vi "Zoe z function.vi"() -> ()   [LabVIEW 2014]
uses:
  <vilib>/vision/NI_Vision_Development_Module.lvlib
panel:
  out "Z Estimation":sgl(graph)
  out "Stage Position":dbl(graph)
  out "Segmented Particle":T1(plugin-control)
  out "COM Y":dbl(graph)
  out "COM X":dbl(graph)
  in  "Stage Position":dbl
  out "Cropped ROI":T1(plugin-control)
  in  "CrossCorrelation RADIUS":dbl
  in  "Template Path":path
  in  "Template Path  2":path
  out "Computational time (s)":dbl
  out "THIS ROI":T1(plugin-control)
  out "Original Image":T1(plugin-control)
  out "Y Centroid":sgl
  out "X Centroid":sgl
  in  "Reset Crop":bool
  in  "Crop":bool
  in  "ROI RADIUS":dbl
  in  "File Path":path
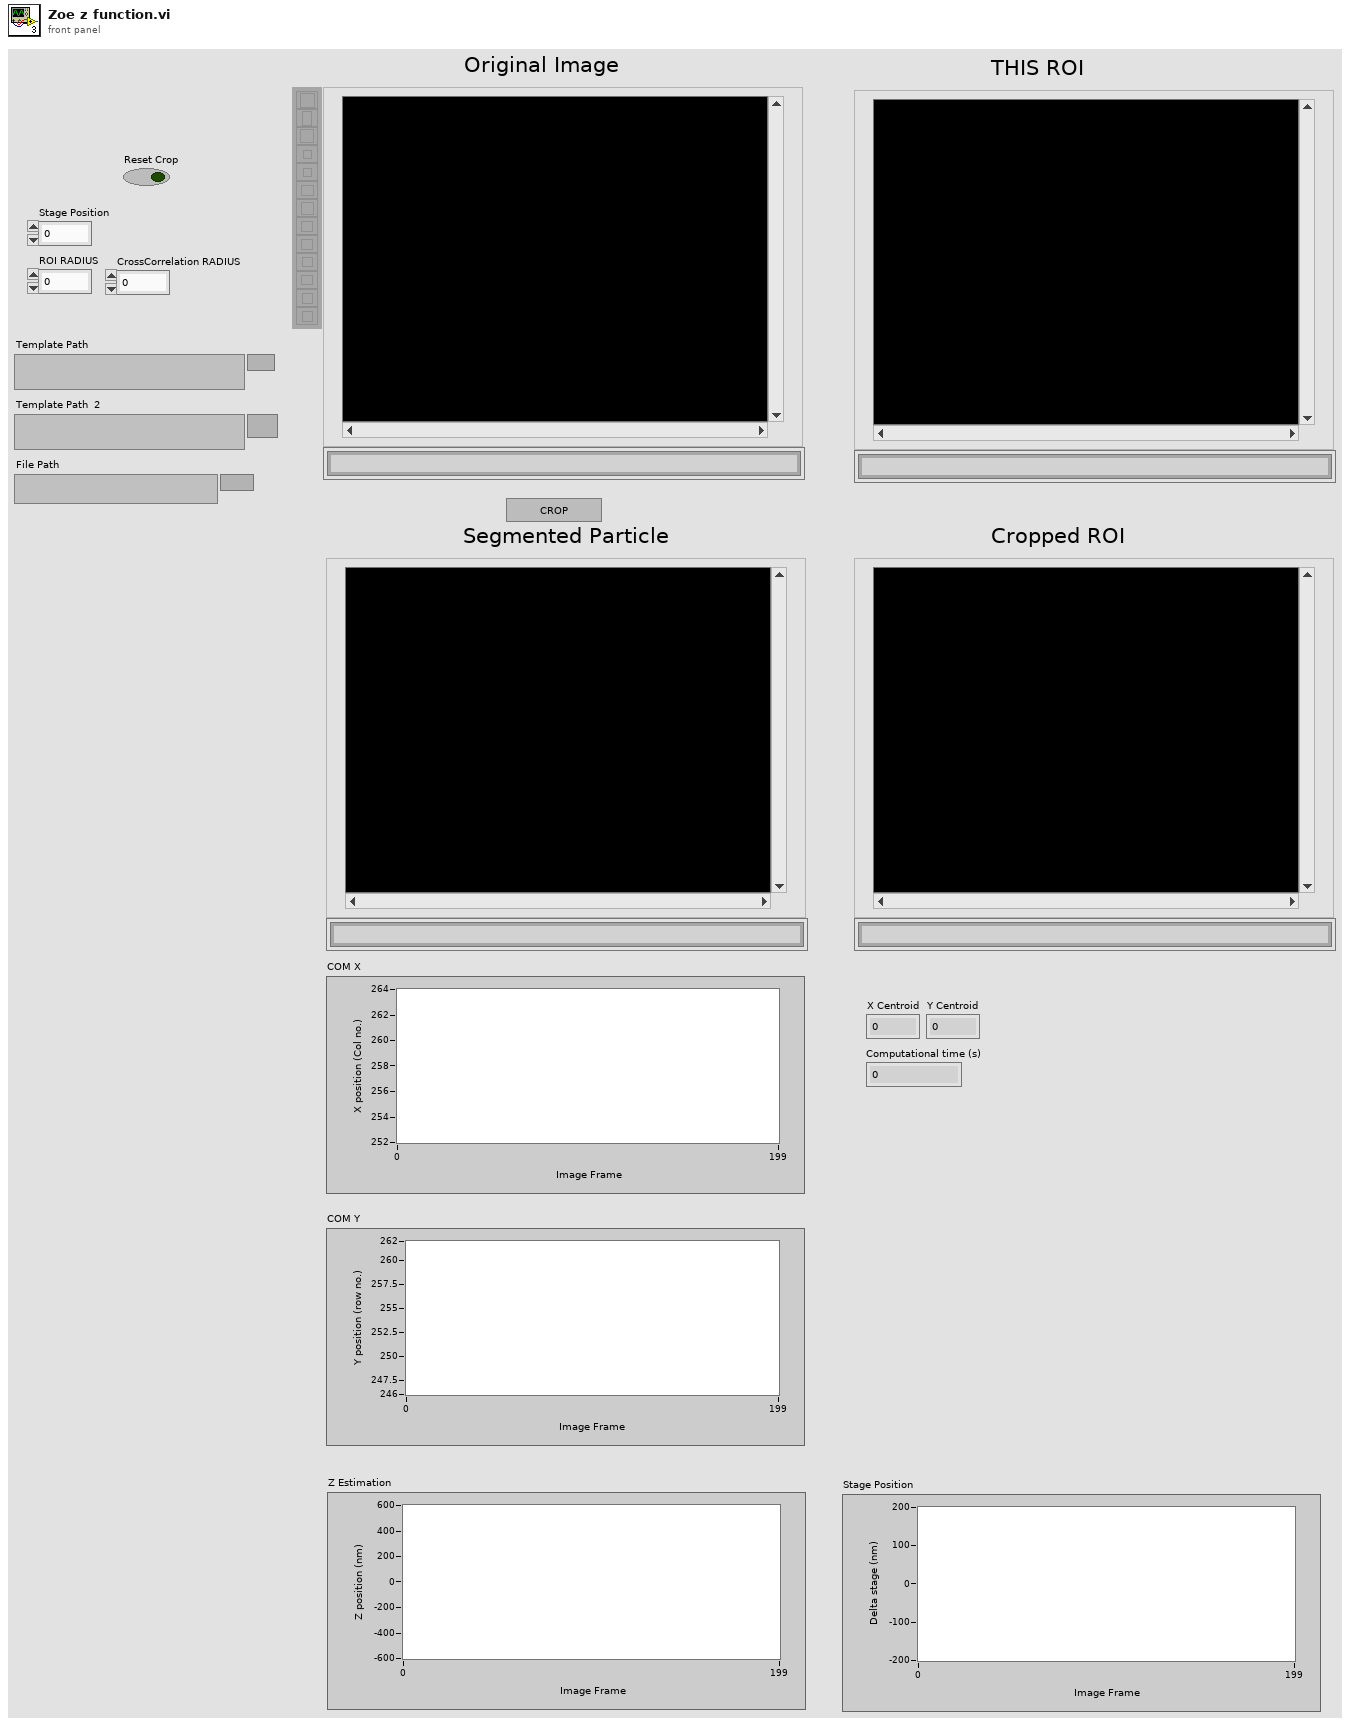
[diagram p1: front panel]
types:
  T1 = typedef "IMAQ Image.ctl" = refnum<image>
  T2 = typedef "Image Type" = u32
  T3 = cluster{"Global Rectangle":i32[], "Contours":cluster{"Contour Type":u32, "ROI Type":u32, "Points":i32[]}[]}
  T4 = typedef "IMAQ Rectangle" = cluster{"Left":i32, "Top":i32, "Right":i32, "Bottom":i32, "Rotation":dbl}
  T5 = cluster{"Mean Value":sgl, "Standard Variation":sgl, "Minimal Value":sgl, "Maximal Value":sgl, "Area (calibrated)":sgl, "Area (pixels)":u32, "%":sgl, "Calibration Valid":bool}
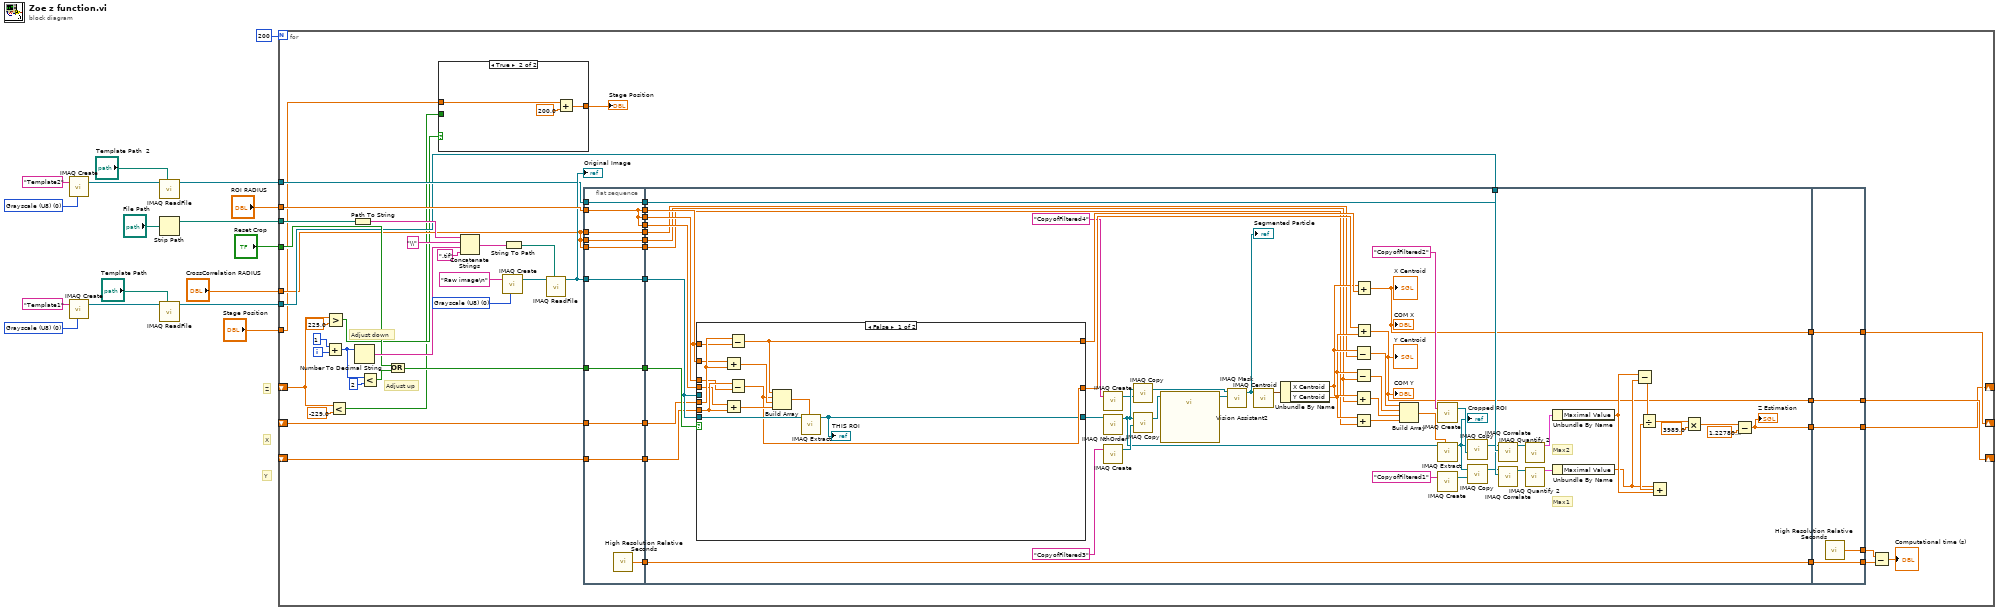
[diagram p0: block diagram]
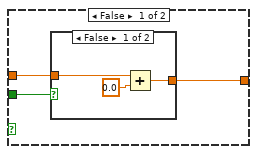
[diagram p2: hidden frame]
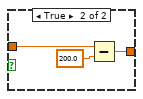
[diagram p3: hidden frame]
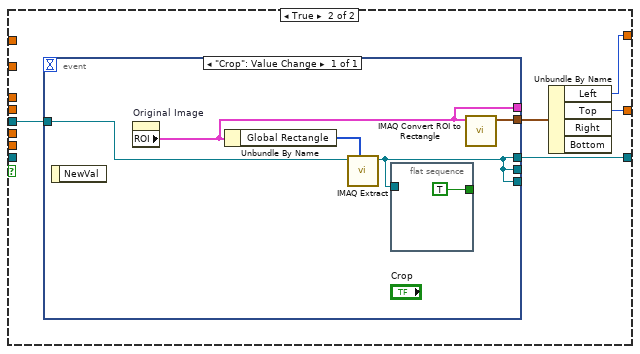
[diagram p4: hidden frame]
diagram:
  w4 = T2 0 items=["Grayscale (U8)", "Grayscale (I16)", "Grayscale (SGL)", "Complex (CSG)", "RGB (U32)", "HSL (U32)", "RGB (U64)", "Grayscale (U16)"] ("Image Type")
  w9 = T2 0 items=["Grayscale (U8)", "Grayscale (I16)", "Grayscale (SGL)", "Complex (CSG)", "RGB (U32)", "HSL (U32)", "RGB (U64)", "Grayscale (U16)"] ("Image Type")
  # "Z"
  # "X"
  # "Y"
  n1 = call "IMAQ Create"("Image Name"="Template2", "Image Type"=w9) -> ("New Image"=w11:T1)  [unwired: 3 in, 1 out]
  n2 = call "IMAQ Create"("Image Name"="Template1", "Image Type"=w4) -> ("New Image"=w6:T1)  [unwired: 3 in, 1 out]
  n3 = call "IMAQ ReadFile"("File Path"="Template Path  2", "Image"=w11) -> ("Image Out"=w8:T1)  [unwired: 5 in, 4 out]
  n4 = Strip Path(path="File Path") -> (stripped path=w14:path)  [unwired: 1 out]
  n5 = call "IMAQ ReadFile"("File Path"="Template Path", "Image"=w6) -> ("Image Out"=w3:T1)  [unwired: 5 in, 4 out]
  n6 = for {
    N: 200 -> [_]
    tunnel: "Reset Crop" -> [w41]
    shift-right: [w64] -> _
    shift-left: _ -> [w61]
    shift-right: [w66] -> _
    shift-left: _ -> [w59]
    tunnel: "ROI RADIUS" -> [w55]
    tunnel: w14 -> [w54]
    tunnel: w8 -> [w35]
    tunnel: w3 -> [w34]
    tunnel: "CrossCorrelation RADIUS" -> [w29]
    shift-right: [w20] -> _
    shift-left: _ -> [w24]
    tunnel: "Stage Position" -> [w21]
    i -> [w46]
    w48 = T2 0 items=["Grayscale (U8)", "Grayscale (I16)", "Grayscale (SGL)", "Complex (CSG)", "RGB (U32)", "HSL (U32)", "RGB (U64)", "Grayscale (U16)"] ("Image Type")
    # "Adjust up"
    # "Adjust down"
    n7 = Add(x=1, y=w46) -> (x+y=w40:i32)
    n8 = Greater?(x=w24, y=225.0) -> (0:w23:bool)
    n9 = Less?(x=w24, y=-229.0) -> (x < y?=w22:bool)
    n10 = Path To String(path=w54) -> (string=w53:string)
    n11 = Number To Decimal String(number=w40) -> (decimal integer string=w44:string)  [unwired: 1 in]
    n12 = Less?(x=w40, y=2) -> (x < y?=w38:bool)
    n13 = Or(x=w41, y=w38) -> (x .or. y?=w37:bool)
    n14 = case shown="True" w23 {
      tunnel: [w72 w81] -> w18
      tunnel: w22 -> [w73 _]
      tunnel: w21 -> [w71 w80]
      frame False {
        n15 = case shown="False" w73 {
          tunnel: [w75 w78] -> w72
          tunnel: w71 -> [w74 w77]
          frame False {
            n16 = Add(x=w74, y=0.0) -> (x+y=w75:dbl)
          }
          frame True {
            n17 = Subtract(x=w77, y=200.0) -> (x-y=w78:dbl)
          }
        }
      }
      frame True {
        n18 = Add(x=w80, y=200.0) -> (x+y=w81:dbl)
      }
    }
    "Stage Position" <- w18
    n19 = Concatenate Strings(w53, "\\" ("string"), w44, ".tif" ("string")) -> (w52:string)
    n20 = call "IMAQ Create"("Image Name"="Raw image\n", "Image Type"=w48) -> ("New Image"=w47:T1)  [unwired: 3 in, 1 out]
    n21 = String To Path(string=w52) -> (path=w51:path)
    n22 = call "IMAQ ReadFile"("File Path"=w51, "Image"=w47) -> ("Image Out"=w50:T1)  [unwired: 5 in, 4 out]
    "Original Image" <- w50
    n23 = flat-sequence {
      tunnel: w50 -> [w91]
      tunnel: w37 -> [w92]
      tunnel: [w92] -> w70
      tunnel: [w91] -> w69
      tunnel: [w90] -> w68
      tunnel: [w89] -> w62
      tunnel: w61 -> [w89]
      tunnel: [w88] -> w60
      tunnel: w59 -> [w88]
      tunnel: [w87] -> w58
      tunnel: [w87] -> w57
      tunnel: [w87] -> w56
      tunnel: w55 -> [w87]
      tunnel: [w86] -> w36
      tunnel: w35 -> [w86]
      tunnel: [w85] -> w31
      tunnel: w29 -> [w85]
      tunnel: w29 -> [w84]
      tunnel: [w84] -> w30
      tunnel: w29 -> [w83]
      tunnel: [w83] -> w28
      tunnel: w70 -> [w147]
      tunnel: w69 -> [w143]
      tunnel: [w142] -> w67
      tunnel: w68 -> [w142]
      tunnel: [w104] -> w65
      tunnel: [w105] -> w63
      tunnel: w62 -> [w141]
      tunnel: w60 -> [w140]
      tunnel: w58 -> [w139]
      tunnel: w57 -> [w138]
      tunnel: w56 -> [w137]
      tunnel: w36 -> [w136]
      tunnel: w34 -> [w135]
      tunnel: w31 -> [w114]
      tunnel: w30 -> [w108]
      tunnel: w28 -> [w113]
      tunnel: [w93] -> w19
      tunnel: [w176] -> w32
      tunnel: w67 -> [w176]
      tunnel: [w175] -> w33
      tunnel: [w174] -> w66
      tunnel: w65 -> [w174]
      tunnel: [w173] -> w64
      tunnel: w63 -> [w173]
      tunnel: [w172] -> w20
      tunnel: w19 -> [w172]
      frame #0 {
        n24 = call <vilib>:"High Resolution Relative Seconds.vi"() -> ("relative seconds"=w90:dbl)
      }
      frame #1 {
        # "Max2"
        # "Max1"
        n25 = case shown="False" w147 {
          tunnel: w143 -> [_ w165]
          tunnel: [w148 w164] -> w146
          tunnel: [w151 w162] -> w145
          tunnel: [w149 w161] -> w144
          tunnel: w143 -> [w160 _]
          tunnel: w141 -> [w159 _]
          tunnel: w140 -> [w158 _]
          tunnel: w138 -> [w157 _]
          tunnel: w139 -> [w156 _]
          tunnel: w138 -> [w155 _]
          tunnel: w137 -> [w154 _]
          frame False {
            n26 = Add(x=w157, y=w159) -> (x+y=w153:dbl)
            n27 = Add(x=w156, y=w158) -> (x+y=w150:dbl)
            n28 = Subtract(x=w159, y=w155) -> (x-y=w151:dbl)
            n29 = Subtract(x=w158, y=w154) -> (x-y=w149:dbl)
            n30 = Build Array(w151, w149, w153, w150) -> (w152:dbl[])
            n31 = call "IMAQ Extract"("Optional Rectangle"=w152, "Image Src"=w160) -> ("Image Dst Out"=w148:T1)  [unwired: 8 in, 1 out]
            "THIS ROI" <- w148
          }
          frame True {
            n32 = event shown="[0] \"Crop\": Value Change" {
              selector: _ -> [_]
              dyn-events: _ -> [_]
              timeout: _ -> [_]
              tunnel: w165 -> [w170]
              tunnel: [w168] -> _
              tunnel: [w168] -> _
              tunnel: [w167] -> _
              tunnel: [w168] -> w164
              tunnel: [w166] -> w163
              event "Crop": Value Change {
                n33 = event-data() -> ()  [unwired: 1 in, 1 out]
                n34 = property on="Original Image" class="ImageControl"() -> ("ROI"=w167:T3)  [unwired: 2 in, 2 out]
                n35 = Unbundle By Name(w167) -> ("Global Rectangle"=w169:i32[])
                n36 = call "IMAQ Extract"("Optional Rectangle"=w169, "Image Src"=w170) -> ("Image Dst Out"=w168:T1)  [unwired: 8 in, 1 out]
                n37 = flat-sequence {
                  tunnel: [TRUE] -> _
                  tunnel: w168 -> [_]
                  frame #0 {
                  }
                }
                n38 = call "IMAQ Convert ROI to Rectangle"("ROI Descriptor"=w167) -> ("Rectangle"=w166:T4)  [unwired: 8 in, 1 out]
              }
            }
            n39 = Unbundle By Name(w163) -> ("Left"=w162:i32, "Top"=w161:i32)  [unwired: 2 out]
          }
        }
        n40 = call "IMAQ Create"("Image Name"="CopyofFiltered4") -> ("New Image"=w98:T1)  [unwired: 4 in, 1 out]
        n41 = call "IMAQ NthOrder"("Image Src"=w146) -> ("Image Dst Out"=w99:T1)  [unwired: 6 in, 1 out]
        n42 = call "IMAQ Create"("Image Name"="CopyofFiltered3") -> ("New Image"=w103:T1)  [unwired: 4 in, 1 out]
        n43 = call "IMAQ Copy"("Image Dst"=w98, "Image Src"=w99) -> ("Image Dst Out"=w96:T1)  [unwired: 4 in, 1 out]
        n44 = call "IMAQ Copy"("Image Dst"=w103, "Image Src"=w99) -> ("Image Dst Out"=w100:T1)  [unwired: 4 in, 1 out]
        n45 = call "Vision Assistant2"("Image In"=w100) -> ("Image Out"=w101:T1)  [unwired: 25 in, 1 out]
        n46 = call "IMAQ Mask"("Image Mask"=w101, "Image Src"=w96) -> ("Image Dst Out"=w94:T1)  [unwired: 3 in, 1 out]
        "Segmented Particle" <- w94
        n47 = call "IMAQ Centroid"("Image"=w94) -> ("Centroid"=w95:cluster{"X Centroid":sgl, "Y Centroid":sgl})  [unwired: 3 in, 1 out]
        n48 = Unbundle By Name(w95) -> ("X Centroid"=w116:sgl, "Y Centroid"=w115:sgl)
        n49 = Subtract(x=w116, y=w114) -> (x-y=w112:dbl)
        n50 = Subtract(x=w115, y=w108) -> (x-y=w111:dbl)
        n51 = Add(x=w116, y=w108) -> (x+y=w110:dbl)
        n52 = Add(x=w115, y=w113) -> (x+y=w109:dbl)
        n53 = Add(x=w116, y=w145) -> (x+y=w105:dbl)
        "X Centroid" <- w105
        "COM X" <- w105
        n54 = Add(x=w144, y=w115) -> (x+y=w104:dbl)
        "Y Centroid" <- w104
        "COM Y" <- w104
        n55 = Build Array(w112, w111, w110, w109) -> (w107:dbl[])
        n56 = call "IMAQ Create"("Image Name"="CopyofFiltered2") -> ("New Image"=w127:T1)  [unwired: 4 in, 1 out]
        n57 = call "IMAQ Extract"("Optional Rectangle"=w107, "Image Src"=w99) -> ("Image Dst Out"=w106:T1)  [unwired: 8 in, 1 out]
        "Cropped ROI" <- w106
        n58 = call "IMAQ Create"("Image Name"="CopyofFiltered1") -> ("New Image"=w130:T1)  [unwired: 4 in, 1 out]
        n59 = call "IMAQ Copy"("Image Dst"=w127, "Image Src"=w106) -> ("Image Dst Out"=w125:T1)  [unwired: 4 in, 1 out]
        n60 = call "IMAQ Copy"("Image Dst"=w130, "Image Src"=w106) -> ("Image Dst Out"=w128:T1)  [unwired: 4 in, 1 out]
        n61 = call "IMAQ Correlate"("Image Src"=w125, "Image Template"=w136) -> ("Image Dst Out"=w133:T1)  [unwired: 5 in, 1 out]
        n62 = call "IMAQ Correlate"("Image Src"=w128, "Image Template"=w135) -> ("Image Dst Out"=w134:T1)  [unwired: 5 in, 1 out]
        n63 = call "IMAQ Quantify 2"("Image"=w133) -> ("Global Report"=w131:T5)  [unwired: 8 in, 2 out]
        n64 = call "IMAQ Quantify 2"("Image"=w134) -> ("Global Report"=w132:T5)  [unwired: 8 in, 2 out]
        n65 = Unbundle By Name(w131) -> ("Maximal Value"=w120:sgl)
        n66 = Unbundle By Name(w132) -> ("Maximal Value"=w119:sgl)
        n67 = Subtract(x=w120, y=w119) -> (x-y=w124:sgl)
        n68 = Add(x=w119, y=w120) -> (x+y=w123:sgl)
        n69 = Divide(x=w124, y=w123) -> (x/y=w117:sgl)
        n70 = Multiply(x=w117, y=sgl 3989.0) -> (x*y=w121:sgl)
        n71 = Subtract(x=w121, y=sgl 1.2278) -> (x-y=w93:sgl)
        "Z Estimation" <- w93
      }
      frame #2 {
        n72 = call <vilib>:"High Resolution Relative Seconds.vi"() -> ("relative seconds"=w175:dbl)
      }
    }
    n73 = Subtract(x=w33, y=w32) -> (x-y=→"Computational time (s)":dbl)
  }
